vi "test_scd_AcqStop.vi"(8 "error in":errorcluster, 11 "SCD in":refnum<class "SCD.lvclass">) -> (0 "error out":errorcluster, 3 "SCD out":refnum<class "SCD.lvclass">)   [LabVIEW 2023, in "horiba.test.lvlib"]
uses:
  horiba.test.lvlib
  Classes/SCD/SCD.lvclass
  C:/Projects/Horiba/horiba-labview-sdk/Source/Classes/GenericDevice/GenericDevice.lvclass
  Classes/SCD/acqSet.ctl
  1a209038-51a4-4f6a-ac39-8f9a875fcd1b.vi
  d66c61a3-f4bd-4936-baf3-4d77ab6cb5b4.vi
  <vilib>/addons/_JKI Toolkits/Caraya/classes/Assert/Assert Equal Value_Variant.vi
  <vilib>/addons/_JKI Toolkits/Caraya/classes/Test/Test.lvclass
  <vilib>/addons/_JKI Toolkits/Caraya/classes/Assert/Assert.lvclass
  <userlib>/_OpenG.lib/lvdata/lvdata.llb/openg_variant.lvlib
panel:
  # "Connector Pane"
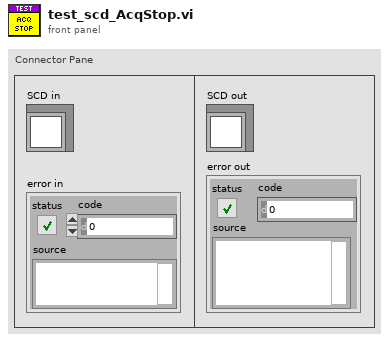
[diagram p1: front panel]
types:
  T1 = typedef "horiba.lvlib/SCD.lvclass/acqSet.ctl" = cluster{"scanCount":i32, "timeStep":i32, "integrationTime":i32, "externalParam":i32}
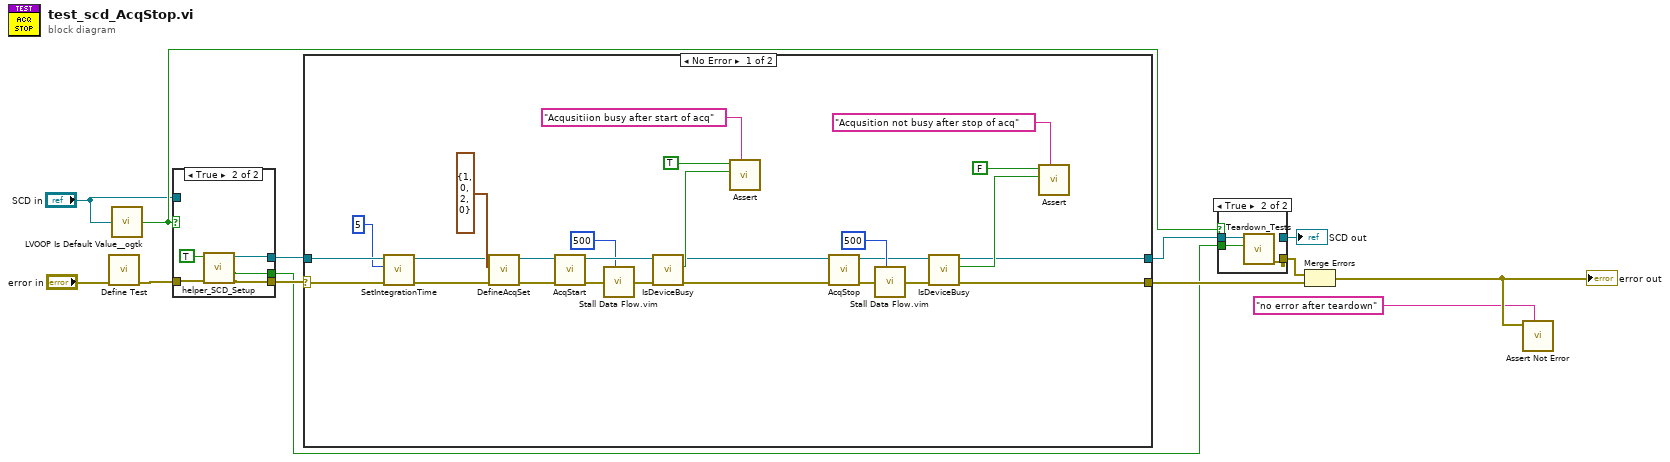
[diagram p0: block diagram]
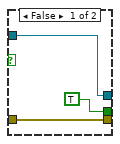
[diagram p2: hidden frame]
diagram:
  n1 = call <vilib>:"Define Test.vi"("error in (no error)"="error in") -> ("error out"=w9:errorcluster)  [unwired: 9 in, 1 out]
  n2 = call <userlib>:"LVOOP Is Default Value__ogtk.vi"("Object"="SCD in") -> ("Is Default Value?"=w3:bool)
  n3 = case shown="True" w3 {
    tunnel: w9 -> [w16 w19]
    tunnel: [w16 w21] -> w8
    tunnel: [w14 w18] -> w7
    tunnel: [TRUE ("Module Was Already Running?") w20] -> w4
    tunnel: "SCD in" -> [w14 _]
    frame False {
    }
    frame True {
      n4 = call "helper_SCD_Setup.vi"("error in"=w19, "show ICL for debugging"=TRUE) -> ("error out"=w21:errorcluster, "Module Was Already Running?"=w20:bool, "SCD out"=w18:refnum<class "SCD.lvclass">)  [unwired: 6 in, 1 out]
    }
  }
  n5 = case shown="No Error" w8 {
    selector: w8 -> [w47 w49]
    tunnel: [w22 w48] -> w12
    tunnel: w7 -> [w35 w48]
    tunnel: [w23 w49] -> w11
    frame No Error {
      n6 = call "SetIntegrationTime.vi"("error in (no error)"=w47, "integration_time"=5, "SCD in"=w35) -> ("error out"=w36:errorcluster, "SCD out"=w34:refnum<class "SCD.lvclass">)  [unwired: 7 in]
      n7 = call "DefineAcqSet.vi"("error in (no error)"=w36, "integration_time"=T1 {"scanCount"=1, "timeStep"=0, "integrationTime"=2, "externalParam"=0}, "SCD in"=w34) -> ("error out"=w45:errorcluster, "SCD out"=w43:refnum<class "SCD.lvclass">)  [unwired: 7 in]
      n8 = call "AcqStart.vi"("error in (no error)"=w45, "SCD in"=w43) -> ("error out"=w44:errorcluster, "SCD out"=w41:refnum<class "SCD.lvclass">)  [unwired: 8 in]
      n9 = call "Stall Data Flow.vim"("value in"=w44, "milliseconds to wait"=u32 500) -> ("value out"=w40:errorcluster)  [unwired: 1 out]
      n10 = call "IsDeviceBusy.vi"("error in (no error)"=w40, "SCD in"=w41) -> ("error out"=w31:errorcluster, "isBusy"=w38:bool, "SCD out"=w32:refnum<class "SCD.lvclass">)  [unwired: 7 in]
      n11 = call-poly <vilib>:"Assert.vi"("Label"="Acqusitiion busy after start of acq", "Y"=w38, "X"=TRUE) -> ()  [unwired: 7 in, 2 out]
      n12 = call "AcqStop.vi"("error in (no error)"=w31, "SCD in"=w32) -> ("error out"=w30:errorcluster, "SCD out"=w28:refnum<class "SCD.lvclass">)  [unwired: 8 in]
      n13 = call "Stall Data Flow.vim"("value in"=w30, "milliseconds to wait"=u32 500) -> ("value out"=w27:errorcluster)  [unwired: 1 out]
      n14 = call "IsDeviceBusy.vi"("error in (no error)"=w27, "SCD in"=w28) -> ("error out"=w23:errorcluster, "isBusy"=w24:bool, "SCD out"=w22:refnum<class "SCD.lvclass">)  [unwired: 7 in]
      n15 = call-poly <vilib>:"Assert.vi"("Label"="Acqusition not busy after stop of acq", "Y"=w24, "X"=FALSE) -> ()  [unwired: 7 in, 2 out]
    }
    frame Error {
    }
  }
  n16 = case shown="True" w3 {
    tunnel: w12 -> [w50 w53]
    tunnel: [_ w52] -> w6
    tunnel: w4 -> [_ w51]
    tunnel: [w50 _] -> w1
    frame False {
    }
    frame True {
      n17 = call "Teardown_Tests.vi"("Module Was Already Running?"=w51, "horiba.lvlib:GenericDevice"=w53) -> ("error out"=w52:errorcluster)  [unwired: 8 in, 1 out]
    }
  }
  "SCD out" <- w1
  n18 = Merge Errors(w6, w11) -> (w10:errorcluster)
  "error out" <- w10
  n19 = call <vilib>:"Assert Not Error.vi"("Label"="no error after teardown", "Not Error?"=w10) -> ()  [unwired: 8 in, 2 out]
